vi "write_to_DAC.vi"(5 "DAC New Reset":bool, 6 "New DAC values generated":T1 {"bit index" min=-1 max=17 step=1; "channel index" max=7 step=1; "offset" max=4095; "DAC voltage"."ch1" max=4095 step=1; "DAC voltage"."ch0" max=4095 step=1}, 7 "DAC values to write In":T1 {"bit index" min=-1 max=17 step=1; "channel index" max=7 step=1; "offset" max=4095; "DAC voltage"."ch1" max=4095 step=1; "DAC voltage"."ch0" max=4095 step=1}, 8 "DAC Reset State In":bool) -> (2 "DAC values to write out":T1 {"bit index" min=-1 max=17 step=1; "channel index" max=7 step=1; "offset" max=4095; "DAC voltage"."ch1" max=4095 step=1; "DAC voltage"."ch0" max=4095 step=1}, 3 "DAC Reset State out":bool)   [LabVIEW 2011]
uses:
  <vilib>/eio/EIONode/EIONode.xnode
  <vilib>/rvi/eio/common/nirviEmuTemplateMethod_errors.vi
  typedefs/DAC_voltage_cluster.ctl
  typedefs/DAC_values_cluster.ctl
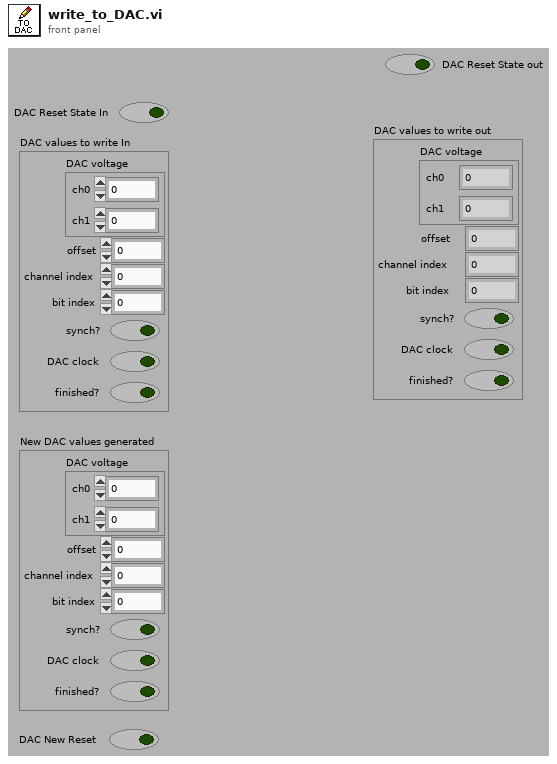
[diagram p1: front panel]
types:
  T1 = typedef "DAC_values_cluster.ctl" = cluster{"DAC voltage":T2, "offset":u16, "channel index":u16, "bit index":i32, "synch?":bool, "DAC clock":bool, "finished?":bool}
  T2 = typedef "DAC_voltage_cluster.ctl" = cluster{"ch0":u16, "ch1":u16}
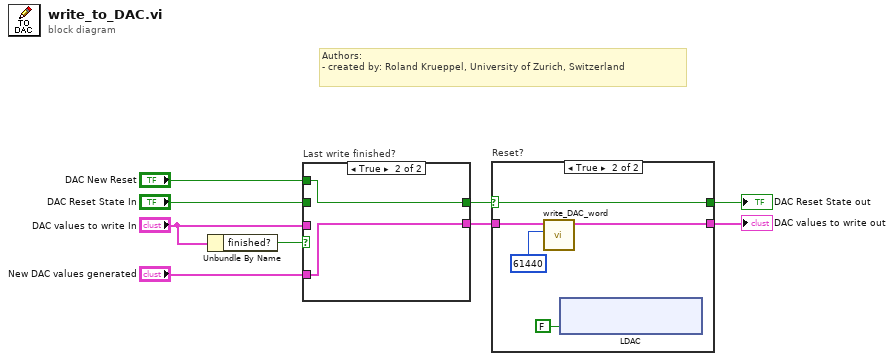
[diagram p0: block diagram]
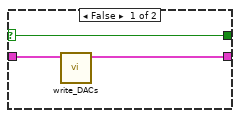
[diagram p2: hidden frame]
diagram:
  # "Authors: \n- created by: Roland Krueppel, University of Zurich, Switzerland"
  n1 = Unbundle By Name("DAC values to write In") -> ("finished?"=w6:bool)
  n2 = case "Last write finished?" shown="True" w6 {
    tunnel: "DAC Reset State In" -> [w10 _]
    tunnel: "DAC values to write In" -> [w11 _]
    tunnel: "New DAC values generated" -> [_ w13]
    tunnel: [w11 w13] -> w3
    tunnel: [w10 w12] -> w2
    tunnel: "DAC New Reset" -> [_ w12]
    frame False {
    }
    frame True {
    }
  }
  n3 = case "Reset?" shown="True" w2 {
    selector: w2 -> [w15 w18]
    tunnel: [w16 w19] -> w4
    tunnel: [w15 w18] -> w5
    tunnel: w3 -> [w14 w17]
    frame False {
      n4 = call "write_DACs.vi"("DAC values in"=w14) -> ("DAQ values out"=w16:T1)  [unwired: 10 in]
    }
    frame True {
      n5 = call "write_DAC_word.vi"("U16 data number"=u16 61440, "DAC values in"=w17) -> ("DAC values out"=w19:T1)  [unwired: 9 in]
      n6 = xnode "LDAC"("Connector1/DIO32"=FALSE ("LDAC")) -> ()  [unwired: 1 in, 1 out]
    }
  }
  "DAC Reset State out" <- w5
  "DAC values to write out" <- w4
